vi "Red_MES.vi"(8 "error in (no error)":errorcluster caption="错误输入（无错误）") -> (0 "error out":errorcluster caption="错误输出", 2 "value":string caption="值")   [LabVIEW 2018]
uses:
  Global.vi
  <vilib>/Utility/config.llb/Read Key (String).vi
  <vilib>/Utility/config.llb/NI_LVConfig.lvlib
panel:
  in  "路径 2":path
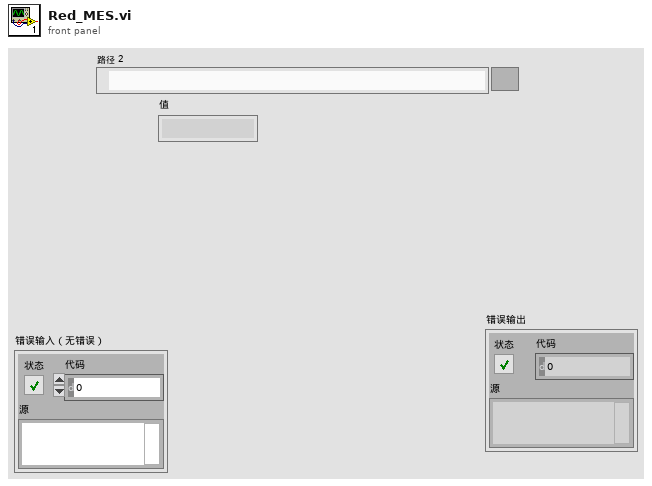
[diagram p1: front panel]
types:
  T1 = typedef "NI_LVConfig.lvlib/Config Data RefNum.ctl" = refnum<k1>
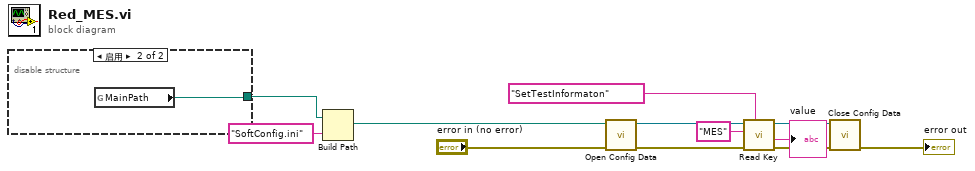
[diagram p0: block diagram]
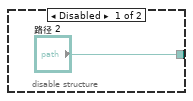
[diagram p2: hidden frame]
diagram:
  n1 = disable-structure shown="启用" {
    disable-tunnel: ["路径 2" w14] -> w11
    frame Disabled {
    }
    frame Enabled {
      n2 = global read "Global.vi" "MainPath"() -> (w14:path)
    }
  }
  n3 = Build Path(base path=w11, name or relative path="SoftConfig.ini" ("名称或相对路径")) -> (appended path=w8:path)
  n4 = call <vilib>:"Open Config Data.vi"("error in (no error)"="error in (no error)", "configuration file path"=w8) -> ("error out"=w5:errorcluster, "refnum"=w6:T1)  [unwired: 7 in, 1 out]
  n5 = call-poly <vilib>:"Read Key.vi"("section"="SetTestInformaton", "error in (no error)"=w5, "key"="MES", "refnum"=w6) -> ("error out"=w3:errorcluster, "value"=→"value":string, "refnum out"=w2:T1)  [unwired: 4 in, 1 out]
  n6 = call <vilib>:"Close Config Data.vi"("error in (no error)"=w3, "refnum"=w2) -> ("error out"=→"error out":errorcluster)  [unwired: 8 in, 1 out]
